vi "Get Label Transfer Config Data Refs.vi"(8 "error in":errorcluster, 11 "Device Ref in":T4 format="%.0x") -> (0 "error out":errorcluster, 3 "Device Ref out":T4 format="%.0x", 4 "Label Transfer Config":T1 {"Block Data Refs"."Data Reference" format="%.0x"})   [LabVIEW 2012, in "AIT 429 Engine.lvlib"]
uses:
  <vilib>/NI Veristand/Custom Device API/Custom Device Item Ref.ctl
  RT Controls/Label Transfer Config.ctl
  <vilib>/NI Veristand/Custom Device API/Block Data Reference.ctl
  <vilib>/NI Veristand/Custom Device API/Data Reference.ctl
  <vilib>/NI Veristand/Custom Device API/Data Access Type.ctl
  <vilib>/NI Veristand/Custom Device Tools/Custom Device Utility Library/NI VeriStand - Search for All Items by GUID.vi
  <vilib>/NI Veristand/Custom Device Tools/Custom Device Utility Library/NI VeriStand - Search for Item by GUID.vi
  Shared/Controls and Global/Global.vi
  AIT 429 Engine.lvlib
  <vilib>/NI Veristand/Custom Device API/Custom Device API.lvlib
  ARINC 429 Shared.lvlib
  <vilib>/NI Veristand/Custom Device Tools/Custom Device Utility Library/Custom Device Utility Library.lvlib
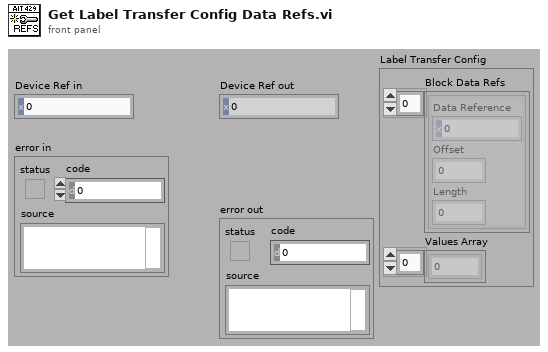
[diagram p1: front panel]
types:
  T1 = typedef "AIT 429 Engine.lvlib/Label Transfer Config.ctl" = cluster{"Block Data Refs":T2[], "Values Array":dbl[]}
  T2 = typedef "Custom Device API.lvlib/Block Data Reference.ctl" = cluster{"Data Reference":T3, "Offset":i32, "Length":i32}
  T3 = typedef "Custom Device API.lvlib/Data Reference.ctl" = i32
  T4 = typedef "Custom Device API.lvlib/Custom Device Item Ref.ctl" = u64
  T5 = typedef "Custom Device API.lvlib/Data Access Type.ctl" = enum16{"Read", "Write"}
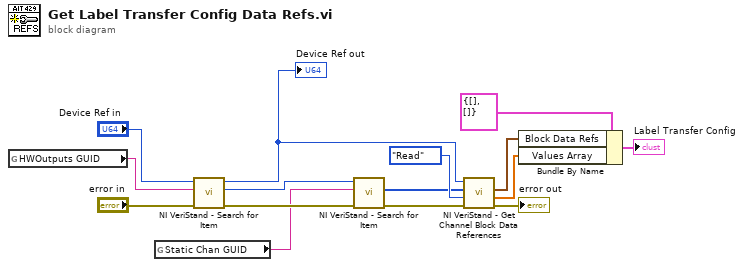
[diagram p0: block diagram]
diagram:
  n1 = global read "Global.vi" "HWOutputs GUID"() -> (w8:string)
  n2 = global read "Global.vi" "Static Chan GUID"() -> (w5:string)
  n3 = call-poly <vilib>:"NI VeriStand - Search for Item.vi"("error in"="error in", "Item GUID"=w8, "Section Ref in"="Device Ref in") -> ("error out"=w7:errorcluster, "Item Ref"=w6:T4, "Section Ref out"=w2:T4)  [unwired: 5 in, 1 out]
  "Device Ref out" <- w2
  n4 = call-poly <vilib>:"NI VeriStand - Search for Item.vi"("error in"=w7, "Item GUID"=w5, "Section Ref in"=w6) -> ("error out"=w4:errorcluster, "Item Refs"=w3:T4[])  [unwired: 5 in, 2 out]
  n5 = call <vilib>:"NI VeriStand - Get Channel Block Data References.vi"("error in (no error)"=w4, "Access"=Data_Access_Type."Read", "Channel Refs"=w3, "Device Ref in"=w2) -> ("error out"=→"error out":errorcluster, "Values Array"=w11:dbl[], "Block Data Refs"=w12:T2[])  [unwired: 4 in, 1 out]
  n6 = Bundle By Name(cluster=T1 {"Block Data Refs"=[], "Values Array"=[]} ("Trans Config"), "Block Data Refs"=w12, "Values Array"=w11) -> (→"Label Transfer Config":T1)
